vi "motorIMU_csvReader_old2.vi"() -> ()   [LabVIEW 2018]
uses:
  Control 12.ctl
  <vilib>/Instr/_visa.llb/VISA Configure Serial Port (Instr).vi
panel:
  in  "Tab Control":enum32{"VISA Config", "IMU", "Motor", "Errors"}(tab)
  in  "VISA":T1="COM4"
  in  "Timeout":u32=10000
  in  "termination char\n(0xA = '\\n' = LF)":u8 format="%.0x"
  in  "Enable Termination\nChar":bool=TRUE
  in  "data bits (8)":u16=8 min=5 max=8 step=1
  in  "parity (0:none)":enum16{"None", "Odd", "Even", "Mark", "Space"}(ring)
  in  "baud rate":u32=115200
  in  "y 2":bool
  in  "stop bits (10: 1 bit)":u16(ring)=10 items=["1.0"=10, "1.5"=15, "2.0"=20]
  out "Temperatura (ºC)":dbl(slide) scale=0.0..50.0 scale format="%#.2f"
  out "Acceleròmetre":cluster{dbl, dbl, dbl}(graph)={-1477.92, 1162.76, -1186.5} caption="Waveform Chart - Dark"
  out "Giroscòpi":cluster{dbl, dbl, dbl}(graph)={-1477.92, 1162.76, -1186.5} caption="Waveform Chart - Dark"
  out "Magnetometre":cluster{dbl, dbl, dbl}(graph)={-4031.37, -986.16, -4204.69} caption="Waveform Chart - Dark"
  in  "y":bool
  in  "y 4":bool
  out "all":string
  out "Bobina 3":bool
  out "Bobina 2":bool
  out "Bobina 1":bool
  out "Motor":cluster{"Data Out":dbl, "Data Out":dbl}(graph) caption="Waveform Chart - Dark"
  in  "y 3":bool
  out "Motor DataString":string
  out "Initial DataString":string
  out "error out":errorcluster
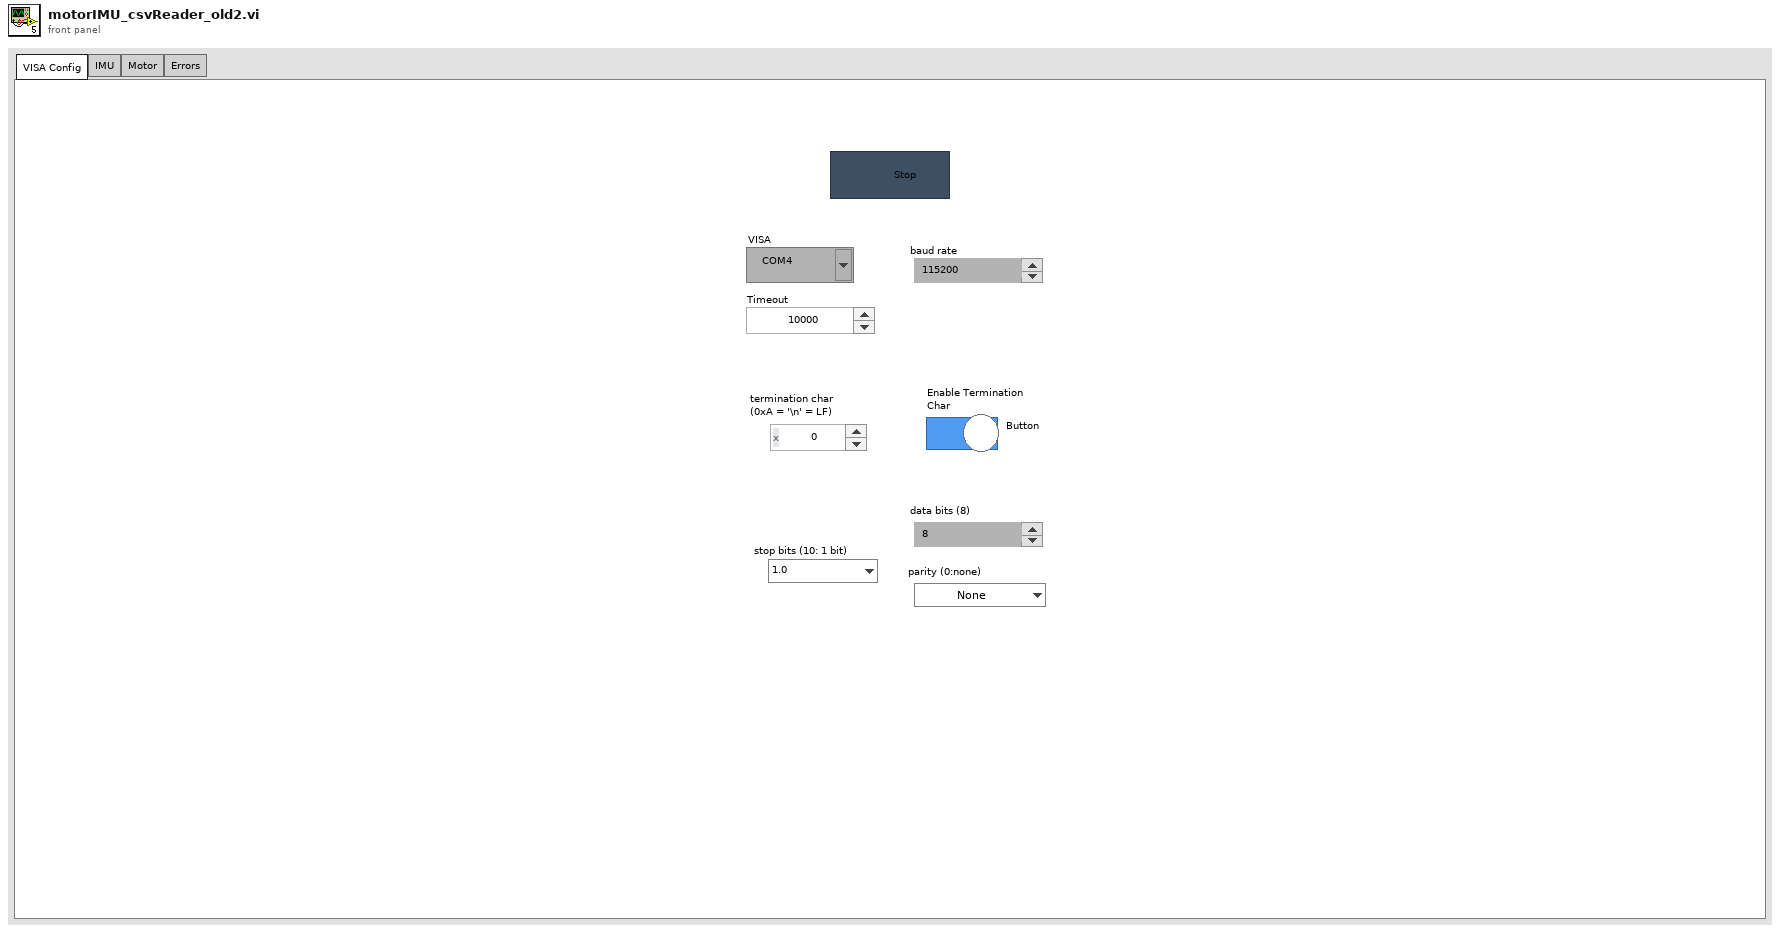
[diagram p1: front panel]
types:
  T1 = typedef "Control 12.ctl" = refnum<visa-resource-name>
  T2 = cluster{"Angle (graus)":dbl, "Fase (#bobina)":dbl}
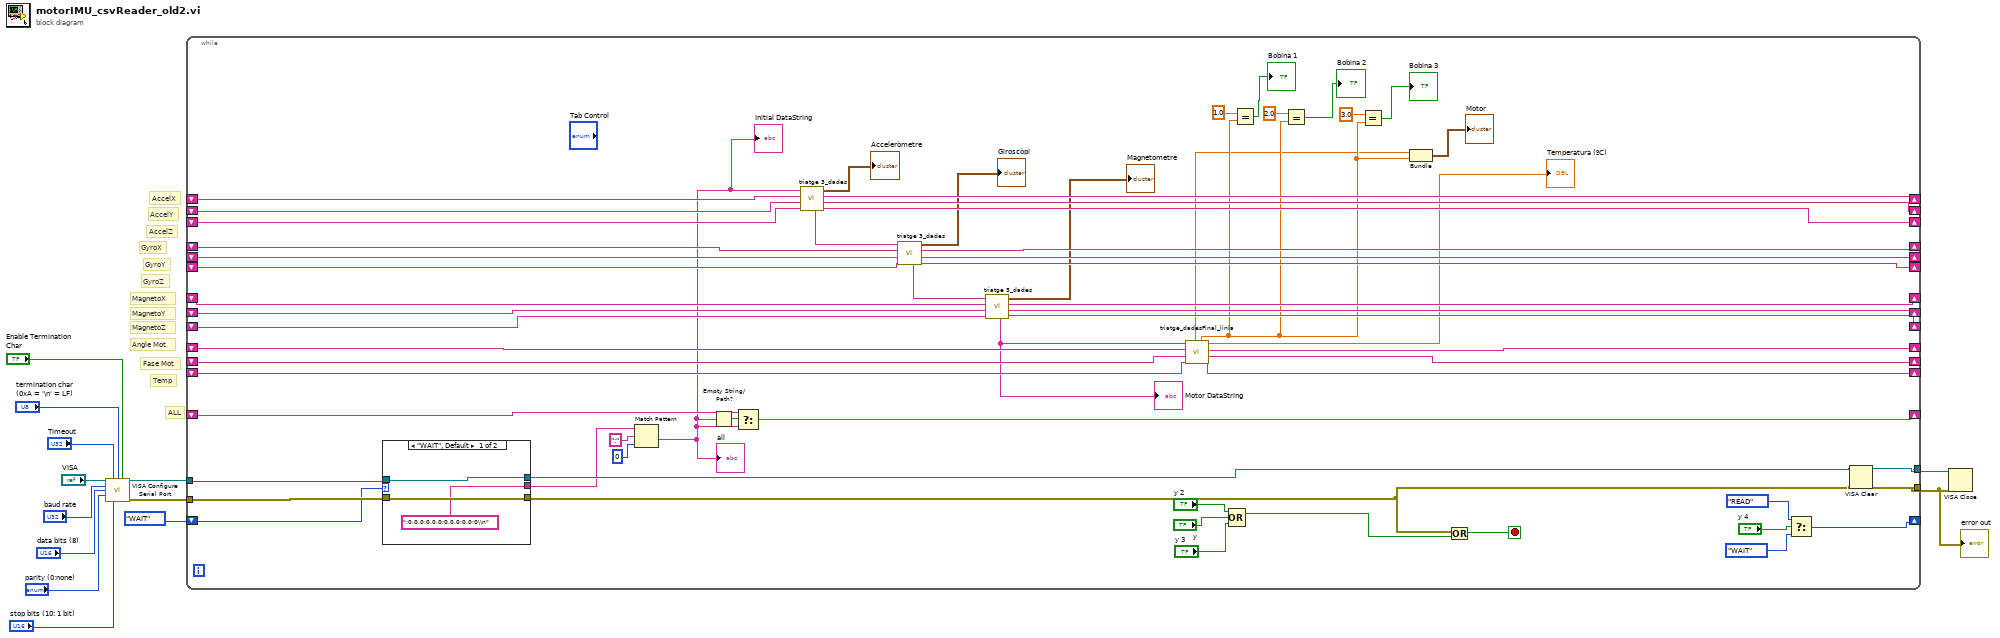
[diagram p0: block diagram]
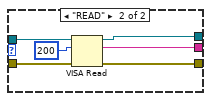
[diagram p2: hidden frame]
diagram:
  # "Fase Mot"
  # "Angle Mot"
  # "ALL"
  # "Temp"
  # "MagnetoZ"
  # "MagnetoY"
  # "MagnetoX"
  # "GyroZ"
  # "AccelZ"
  # "GyroY"
  # "AccelY"
  # "GyroX"
  # "AccelX"
  n1 = call-poly "VISA Configure Serial Port"("VISA resource name"="VISA", "timeout (10sec)"="Timeout", "termination char\n(0xA = '\\n' = LF)"="termination char\n(0xA = '\\n' = LF)", "Enable Termination\nChar (T)"="Enable Termination\nChar", "baud rate (9600)"="baud rate", "data bits (8)"="data bits (8)", "parity (0:none)"="parity (0:none)", "stop bits (10: 1 bit)"="stop bits (10: 1 bit)") -> ("VISA resource name out"=w1:refnum<visa-resource-name>, "error out"=w2:errorcluster)  [unwired: 6 in]
  n2 = while {
    tunnel: [w76] -> w14
    tunnel: [w71] -> w13
    shift-right: [w56] -> _
    shift-left: _ -> [w57]
    shift-right: [w54] -> _
    shift-left: _ -> [w55]
    shift-right: [w44] -> _
    shift-left: _ -> [w45]
    shift-right: [w48] -> _
    shift-left: _ -> [w49]
    shift-right: [w46] -> _
    shift-left: _ -> [w47]
    shift-right: [w52] -> _
    shift-left: _ -> [w53]
    shift-right: [w36] -> _
    shift-left: _ -> [w37]
    shift-right: [w38] -> _
    shift-left: _ -> [w39]
    shift-right: [w40] -> _
    shift-left: _ -> [w41]
    shift-right: [w50] -> _
    shift-left: _ -> [w66]
    shift-right: [w35] -> _
    shift-left: _ -> [w34]
    shift-right: [w30] -> _
    shift-left: _ -> [w31]
    shift-right: [w33] -> _
    shift-left: _ -> [w32]
    shift-right: [w22] -> _
    shift-left: enum16{"WAIT", "READ", ""}."WAIT" -> [w16]
    tunnel: w2 -> [w18]
    tunnel: w1 -> [w17]
    stop <- w72 stop-if-true
    n3 = case shown="\"WAIT\", Default" w16 {
      tunnel: [w79 w84] -> w76
      tunnel: [":0,0,0;0,0,0;0,0,0;0,0;0\\n" w83] -> w73
      tunnel: [w78 w82] -> w71
      tunnel: w17 -> [w79 w81]
      tunnel: w18 -> [w78 w80]
      frame "WAIT", Default {
      }
      frame "READ" {
        n4 = VISA Read(VISA resource name=w81, byte count=u32 200, error in (no error)=w80) -> (VISA resource name out=w84:refnum<visa-resource-name>, read buffer=w83:string, error out=w82:errorcluster)  [unwired: 1 out]
      }
    }
    n5 = Match Pattern(string=w73, regular expression=":", offset (0)=0 ("t")) -> (after substring=w24:string)  [unwired: 3 out]
    "Initial DataString" <- w24
    "all" <- w24
    n6 = Empty String/Path?(string/path=w24) -> (empty?=w67:bool)
    n7 = Select(t=w66, s=w67, f=w24) -> (s? t:f=w50:string)
    n8 = call "triatge 3_dades.vi"("shift register left 3"=w53, "shift register left 2"=w55, "shift register left"=w57, "DataIN"=w24) -> ("shift register right 3"=w52:string, "shift register right 2"=w54:string, "shift register right"=w56:string, "Acceleròmetre"=→"Acceleròmetre":cluster{dbl, dbl, dbl}, "String Out"=w42:string)  [unwired: 3 in]
    n9 = call "triatge 3_dades.vi"("shift register left 3"=w45, "shift register left 2"=w47, "shift register left"=w49, "DataIN"=w42) -> ("shift register right 3"=w44:string, "shift register right 2"=w46:string, "shift register right"=w48:string, "Acceleròmetre"=→"Giroscòpi":cluster{dbl, dbl, dbl}, "String Out"=w23:string)  [unwired: 3 in]
    n10 = call "triatge 3_dades.vi"("shift register left 3"=w37, "shift register left 2"=w39, "shift register left"=w41, "DataIN"=w23) -> ("shift register right 3"=w36:string, "shift register right 2"=w38:string, "shift register right"=w40:string, "Acceleròmetre"=→"Magnetometre":cluster{dbl, dbl, dbl}, "String Out"=w25:string)  [unwired: 3 in]
    "Motor DataString" <- w25
    n11 = call "triatge_dadesFinal_linia.vi"("shift register left 3"=w31, "shift register left 2"=w32, "shift register left"=w34, "String in"=w25) -> ("shift register right 3"=w30:string, "shift register right 2"=w33:string, "shift register right"=w35:string, "Temp"=→"Temperatura (ºC)":dbl, "Fase (#bobina)"=w29:dbl, "Angle (graus)"=w28:dbl)  [unwired: 2 in]
    n12 = Compound Arithmetic op=OR("y 2", "y", "y 3") -> (w68:bool)
    n13 = Equal?(x=1.0, y=w29) -> (x = y?=→"Bobina 1":bool)
    n14 = Equal?(x=2.0, y=w29) -> (x = y?=→"Bobina 2":bool)
    n15 = Equal?(x=3.0, y=w29) -> (x = y?=→"Bobina 3":bool)
    n16 = Bundle("Angle (graus)"=w28, "Fase (#bobina)"=w29) -> (→"Motor":T2)  [unwired: 1 in]
    n17 = Or(x=w71, y=w68) -> (x .or. y?=w72:bool)
    n18 = Select(t=enum16{"WAIT", "READ", ""}."READ", s="y 4", f=enum16{"WAIT", "READ", ""}."WAIT") -> (s? t:f=w22:enum16{"WAIT", "READ", ""})
  }
  n19 = VISA Clear(VISA resource name=w14, error in (no error)=w13) -> (VISA resource name out=w15:refnum<visa-resource-name>, error out=w12:errorcluster)
  "error out" <- w12
  n20 = VISA Close(VISA resource name=w15, error in (no error)=w12) -> ()  [unwired: 1 out]
